vi "Route Triggers Gain Ranging.vi"(0 "pxi trigger bus configuration [channel]":T1[](array[typedef]), 1 "scope":string, 2 "map(T)/unmap(F)":bool=TRUE, 5 "routing mode":enum16{"Master Channel", "Independent Channels"}(ring), 11 "error in":errorcluster, 13 "gain config PXI triggers [channel]":string[][](array[combo])=[["None"], ["None"]], 14 "mmWave port config PXI trigger [channel]":string[](array[combo])=["None"]) -> (15 "error out":errorcluster)   [LabVIEW 2019]
uses:
  TypeDefs/PXI Trigger Bus Info.ctl
  <instrlib>/niMmWave/ni3620/Config/v1/Host/Public/Typedefs/PXI Trigger.ctl
  <vilib>/Instr/_visa.llb/VISA Unmap Trigger Trigger Source.ctl
  <instrlib>/niMmWave/ni3620/Config/v1/Host/niMmWave Config v1 Host.lvlib
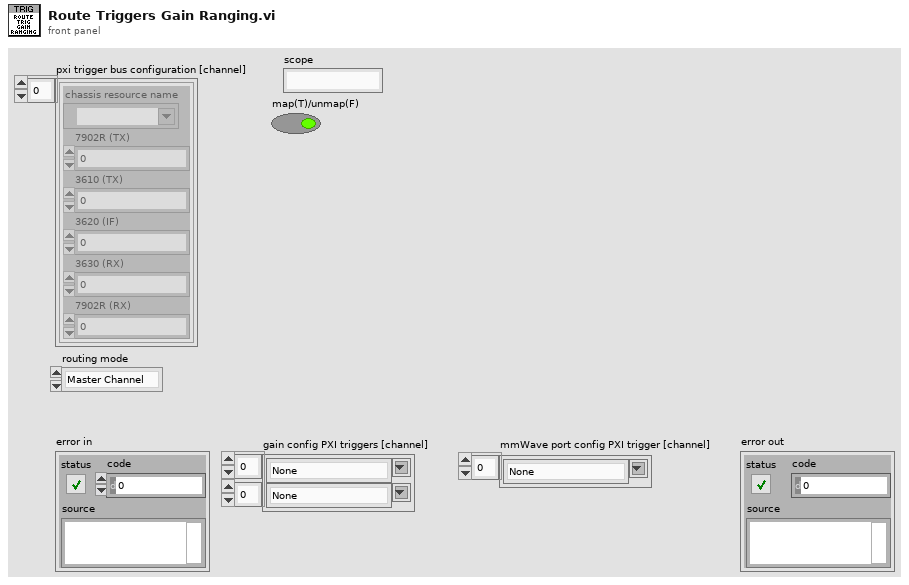
[diagram p1: front panel]
types:
  T1 = typedef "PXI Trigger Bus Info.ctl" = cluster{"chassis resource name":refnum<visa-resource-name>, "7902R (TX)":i16, "3610 (TX)":i16, "3620 (IF)":i16, "3630 (RX)":i16, "7902R (RX)":i16}
  T2 = typedef "niMmWave Config v1 Host.lvlib/PXI Trigger.ctl" = enum16{"PXI_Trig0", "PXI_Trig1", "PXI_Trig2", "PXI_Trig3", "PXI_Trig4", "PXI_Trig5", "PXI_Trig6", "PXI_Trig7", "None"}
  T3 = typedef "VISA Unmap Trigger Trigger Source.ctl" = i16
  T4 = cluster{"chassis":refnum<visa-resource-name>, "pxi trigger number":T3, "source trigger segment":i16, "destination trigger segment":i16}
  T5 = cluster{"chassis":refnum<visa-resource-name>, "pxi trigger number":T3, "source trigger segment":i16, "destination trigger segment":i16}[]
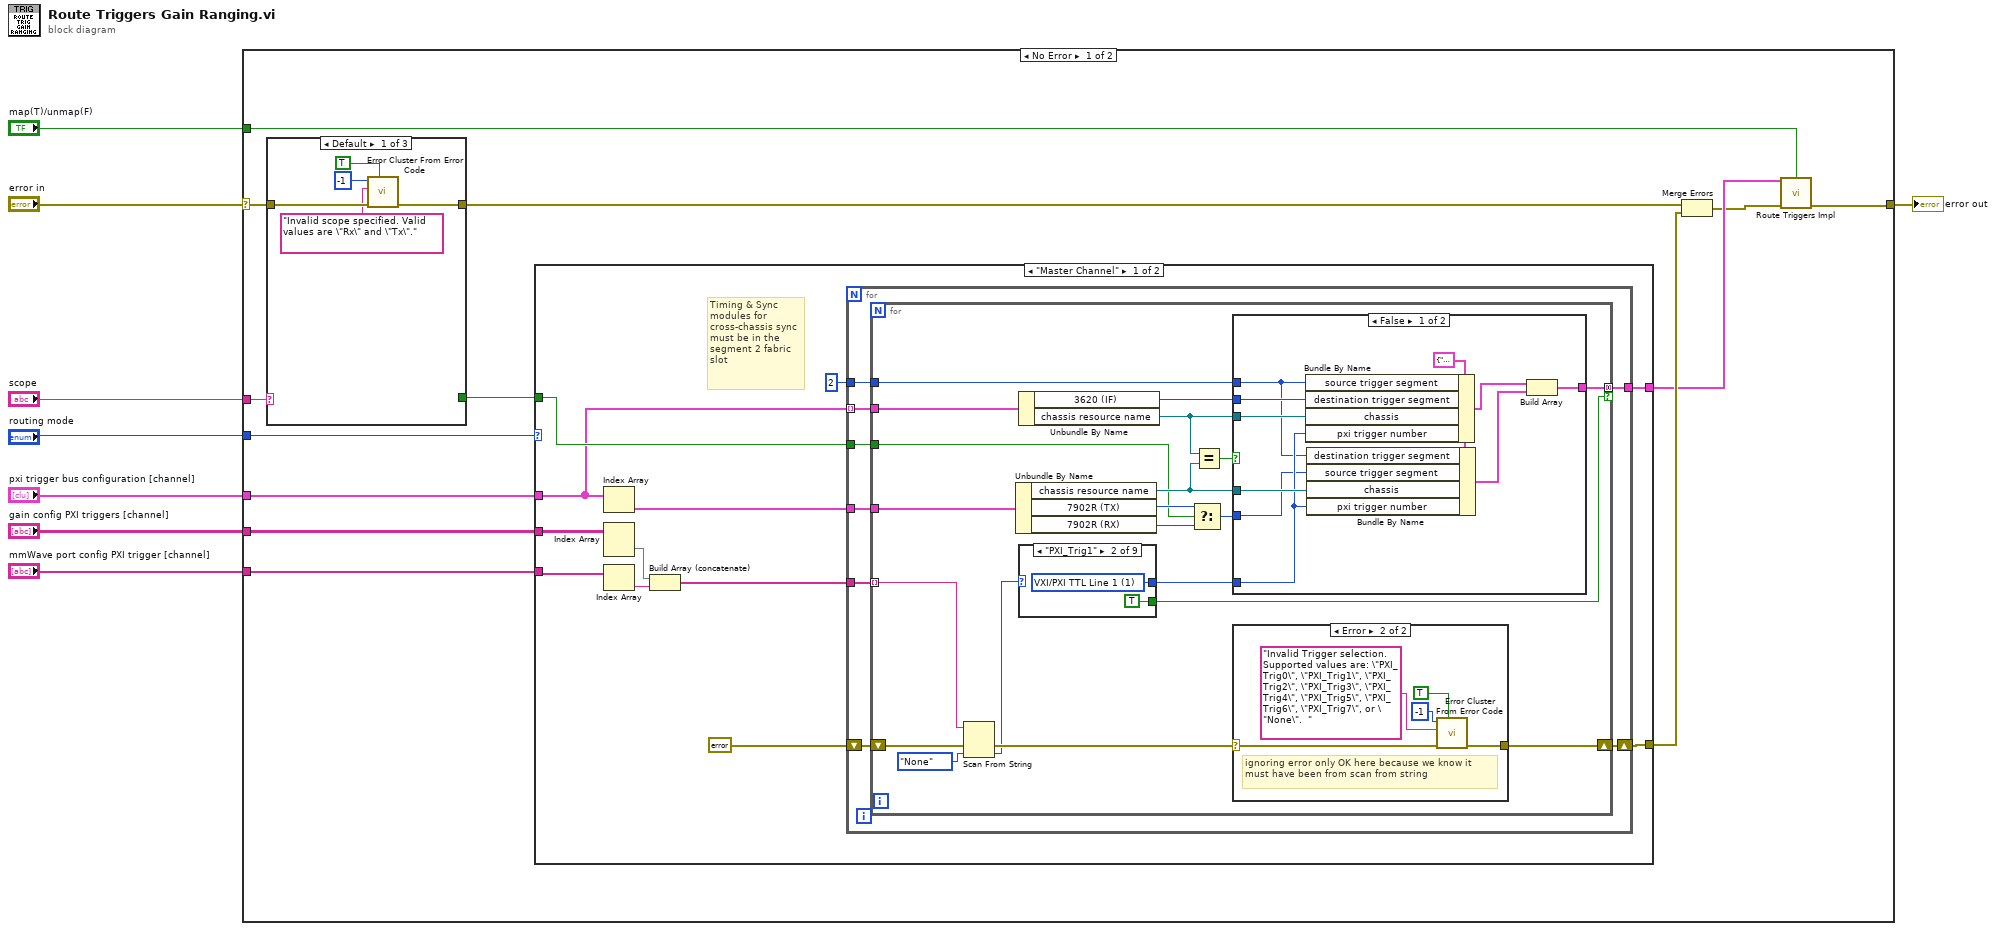
[diagram p0: block diagram]
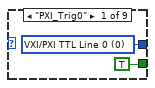
[diagram p3: hidden frame]
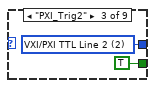
[diagram p4: hidden frame]
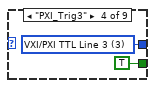
[diagram p5: hidden frame]
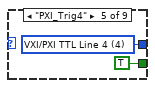
[diagram p6: hidden frame]
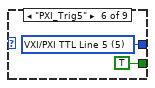
[diagram p7: hidden frame]
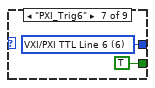
[diagram p8: hidden frame]
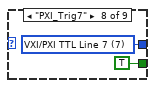
[diagram p9: hidden frame]
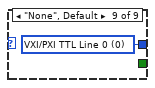
[diagram p10: hidden frame]
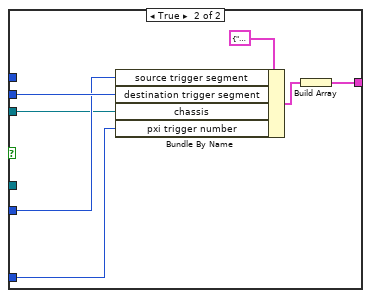
[diagram p11: hidden frame]
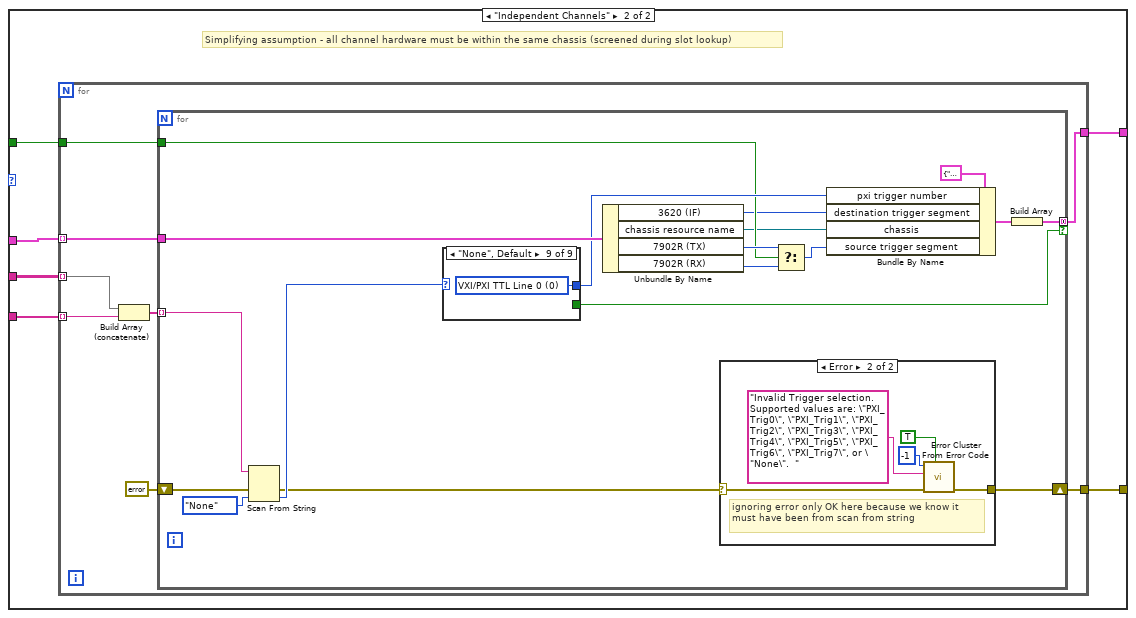
[diagram p12: hidden frame]
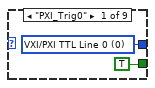
[diagram p14: hidden frame]
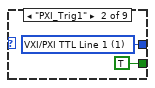
[diagram p15: hidden frame]
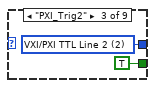
[diagram p16: hidden frame]
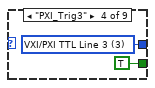
[diagram p17: hidden frame]
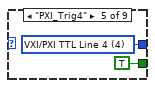
[diagram p18: hidden frame]
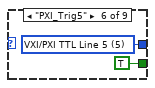
[diagram p19: hidden frame]
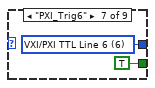
[diagram p20: hidden frame]
diagram:
  n1 = case shown="No Error" "error in" {
    selector: "error in" -> [w20 w166]
    tunnel: [w9 w166] -> w8
    tunnel: "map(T)/unmap(F)" -> [w11 _]
    tunnel: "pxi trigger bus configuration [channel]" -> [w21 _]
    tunnel: "scope" -> [w19 _]
    tunnel: "routing mode" -> [w17 _]
    tunnel: "gain config PXI triggers [channel]" -> [w16 _]
    tunnel: "mmWave port config PXI trigger [channel]" -> [w15 _]
    frame No Error {
      n2 = case shown="Default" w19 {
        tunnel: [w160 w163 w165] -> w14
        tunnel: w20 -> [w161 w163 w165]
        tunnel: [_ FALSE TRUE] -> w18
        frame Default {
          n3 = call <vilib>:"Error Cluster From Error Code.vi"("show call chain? (False)"=TRUE, "error in (no error)"=w161, "error message (\"\")"="Invalid scope specified. Valid values are \"Rx\" and \"Tx\"." ("error message (\"\")"), "error code (0)"=-1) -> ("error out"=w160:errorcluster)  [unwired: 5 in]
        }
        frame "rx" {
        }
        frame "tx" {
        }
      }
      n4 = case shown="\"Master Channel\"" w17 {
        tunnel: w21 -> [w22 w107]
        tunnel: [w33 w106] -> w12
        tunnel: w18 -> [w32 w105]
        tunnel: w16 -> [w29 w104]
        tunnel: w15 -> [w30 w103]
        tunnel: [w23 w102] -> w13
        frame "Master Channel" {
          # "Timing & Sync modules for cross-chassis sync must be in the segment 2 fabric slot"
          n5 = Index Array(array=w22) -> (element=w28:T1)  [unwired: 1 in]
          n6 = Index Array(array=w29) -> (element=w27:string[])  [unwired: 2 in]
          n7 = Index Array(array=w30) -> (element=w26:string)  [unwired: 1 in]
          n8 = Build Array (concatenate)(w27, w26) -> (w25:string[])
          n9 = for {
            tunnel: [w41] -> w33
            tunnel: w32 -> [w40]
            tunnel: i16 2 ("source trigger segment") -> [w39]
            tunnel: w28 -> [w38]
            tunnel: w25 -> [w37]
            tunnel: w22 -> [w34] mode=indexing
            shift-right: [w35] -> w23
            shift-left: errorcluster {"status"=FALSE, "code"=0, "source"=""} ("error out") -> [w36]
            n10 = for {
              tunnel: [w61] -> w41 mode=concatenating if=w43
              tunnel: w40 -> [w53]
              tunnel: w39 -> [w52]
              tunnel: w38 -> [w51]
              tunnel: w37 -> [w47] mode=indexing
              shift-right: [w45] -> w35
              shift-left: w36 -> [w46]
              tunnel: w34 -> [w42]
              n11 = Scan From String(input string=w47, error in=w46, default 1=PXI_Trigger."None" ("PXI Trigger")) -> (error out=w50:errorcluster, output 1=w49:T2)  [unwired: 2 in, 2 out]
              n12 = Unbundle By Name(w51) -> ("chassis resource name"=w59:refnum<visa-resource-name>, "7902R (TX)"=w56:i16, "7902R (RX)"=w55:i16)
              n13 = Unbundle By Name(w42) -> ("3620 (IF)"=w60:i16, "chassis resource name"=w57:refnum<visa-resource-name>)
              n14 = case shown="\"PXI_Trig1\"" w49 {
                tunnel: [w69 w71 w73 w75 w77 w79 w81 w83 w84] -> w44
                tunnel: [TRUE ("x = y?") TRUE ("x = y?") TRUE ("x = y?") TRUE ("x = y?") TRUE ("x = y?") TRUE ("x = y?") TRUE ("x = y?") TRUE ("x = y?") _] -> w43
                frame "PXI_Trig0" {
                  w69 = T3 0 items=["VXI/PXI TTL Line 0"=0, "VXI/PXI TTL Line 1"=1, "VXI/PXI TTL Line 2"=2, "VXI/PXI TTL Line 3"=3, "VXI/PXI TTL Line 4"=4, "VXI/PXI TTL Line 5"=5, "VXI/PXI TTL Line 6"=6, "VXI/PXI TTL Line 7"=7, "VXI ECL Line 0"=8, "VXI ECL Line 1"=9, "Front Panel Input"=27, "Front Panel Output"=28] ("pxi trigger number")
                }
                frame "PXI_Trig1" {
                  w71 = T3 1 items=["VXI/PXI TTL Line 0"=0, "VXI/PXI TTL Line 1"=1, "VXI/PXI TTL Line 2"=2, "VXI/PXI TTL Line 3"=3, "VXI/PXI TTL Line 4"=4, "VXI/PXI TTL Line 5"=5, "VXI/PXI TTL Line 6"=6, "VXI/PXI TTL Line 7"=7, "VXI ECL Line 0"=8, "VXI ECL Line 1"=9, "Front Panel Input"=27, "Front Panel Output"=28] ("pxi trigger number")
                }
                frame "PXI_Trig2" {
                  w73 = T3 2 items=["VXI/PXI TTL Line 0"=0, "VXI/PXI TTL Line 1"=1, "VXI/PXI TTL Line 2"=2, "VXI/PXI TTL Line 3"=3, "VXI/PXI TTL Line 4"=4, "VXI/PXI TTL Line 5"=5, "VXI/PXI TTL Line 6"=6, "VXI/PXI TTL Line 7"=7, "VXI ECL Line 0"=8, "VXI ECL Line 1"=9, "Front Panel Input"=27, "Front Panel Output"=28] ("pxi trigger number")
                }
                frame "PXI_Trig3" {
                  w75 = T3 3 items=["VXI/PXI TTL Line 0"=0, "VXI/PXI TTL Line 1"=1, "VXI/PXI TTL Line 2"=2, "VXI/PXI TTL Line 3"=3, "VXI/PXI TTL Line 4"=4, "VXI/PXI TTL Line 5"=5, "VXI/PXI TTL Line 6"=6, "VXI/PXI TTL Line 7"=7, "VXI ECL Line 0"=8, "VXI ECL Line 1"=9, "Front Panel Input"=27, "Front Panel Output"=28] ("pxi trigger number")
                }
                frame "PXI_Trig4" {
                  w77 = T3 4 items=["VXI/PXI TTL Line 0"=0, "VXI/PXI TTL Line 1"=1, "VXI/PXI TTL Line 2"=2, "VXI/PXI TTL Line 3"=3, "VXI/PXI TTL Line 4"=4, "VXI/PXI TTL Line 5"=5, "VXI/PXI TTL Line 6"=6, "VXI/PXI TTL Line 7"=7, "VXI ECL Line 0"=8, "VXI ECL Line 1"=9, "Front Panel Input"=27, "Front Panel Output"=28] ("pxi trigger number")
                }
                frame "PXI_Trig5" {
                  w79 = T3 5 items=["VXI/PXI TTL Line 0"=0, "VXI/PXI TTL Line 1"=1, "VXI/PXI TTL Line 2"=2, "VXI/PXI TTL Line 3"=3, "VXI/PXI TTL Line 4"=4, "VXI/PXI TTL Line 5"=5, "VXI/PXI TTL Line 6"=6, "VXI/PXI TTL Line 7"=7, "VXI ECL Line 0"=8, "VXI ECL Line 1"=9, "Front Panel Input"=27, "Front Panel Output"=28] ("pxi trigger number")
                }
                frame "PXI_Trig6" {
                  w81 = T3 6 items=["VXI/PXI TTL Line 0"=0, "VXI/PXI TTL Line 1"=1, "VXI/PXI TTL Line 2"=2, "VXI/PXI TTL Line 3"=3, "VXI/PXI TTL Line 4"=4, "VXI/PXI TTL Line 5"=5, "VXI/PXI TTL Line 6"=6, "VXI/PXI TTL Line 7"=7, "VXI ECL Line 0"=8, "VXI ECL Line 1"=9, "Front Panel Input"=27, "Front Panel Output"=28] ("pxi trigger number")
                }
                frame "PXI_Trig7" {
                  w83 = T3 7 items=["VXI/PXI TTL Line 0"=0, "VXI/PXI TTL Line 1"=1, "VXI/PXI TTL Line 2"=2, "VXI/PXI TTL Line 3"=3, "VXI/PXI TTL Line 4"=4, "VXI/PXI TTL Line 5"=5, "VXI/PXI TTL Line 6"=6, "VXI/PXI TTL Line 7"=7, "VXI ECL Line 0"=8, "VXI ECL Line 1"=9, "Front Panel Input"=27, "Front Panel Output"=28] ("pxi trigger number")
                }
                frame "None", Default {
                  w84 = T3 0 items=["VXI/PXI TTL Line 0"=0, "VXI/PXI TTL Line 1"=1, "VXI/PXI TTL Line 2"=2, "VXI/PXI TTL Line 3"=3, "VXI/PXI TTL Line 4"=4, "VXI/PXI TTL Line 5"=5, "VXI/PXI TTL Line 6"=6, "VXI/PXI TTL Line 7"=7, "VXI ECL Line 0"=8, "VXI ECL Line 1"=9, "Front Panel Input"=27, "Front Panel Output"=28] ("pxi trigger number")
                }
              }
              n15 = Select(t=w56, s=w53, f=w55) -> (s? t:f=w54:i16)
              n16 = Equal?(x=w57, y=w59) -> (x = y?=w58:bool)
              n17 = case shown="False" w58 {
                tunnel: [w93 w100] -> w61
                tunnel: w60 -> [w92 w98]
                tunnel: w59 -> [w89 _]
                tunnel: w57 -> [w91 w95]
                tunnel: w52 -> [w85 _]
                tunnel: w54 -> [w86 w97]
                tunnel: w44 -> [w87 w96]
                frame False {
                  w90 = T4 {"chassis"="", "pxi trigger number"=0, "source trigger segment"=0, "destination trigger segment"=0} ("Trigger Route")
                  n18 = Bundle By Name(cluster=w90, "source trigger segment"=w85, "destination trigger segment"=w92, "chassis"=w91, "pxi trigger number"=w87) -> (w94:T4)
                  n19 = Bundle By Name(cluster=w90, "destination trigger segment"=w85, "source trigger segment"=w86, "chassis"=w89, "pxi trigger number"=w87) -> (w88:T4)
                  n20 = Build Array(w94, w88) -> (w93:T5)
                }
                frame True {
                  n21 = Bundle By Name(cluster=T4 {"chassis"="", "pxi trigger number"=0, "source trigger segment"=0, "destination trigger segment"=0} ("Trigger Route"), "source trigger segment"=w97, "destination trigger segment"=w98, "chassis"=w95, "pxi trigger number"=w96) -> (w101:T4)
                  n22 = Build Array(w101) -> (w100:T5)
                }
              }
              n23 = case shown="Error" w50 {
                selector: w50 -> [w62 w63]
                tunnel: [w62 w64] -> w45
                frame No Error {
                }
                frame Error {
                  # "ignoring error only OK here because we know it must have been from scan from string"
                  n24 = call <vilib>:"Error Cluster From Error Code.vi"("show call chain? (False)"=TRUE, "error in (no error)"=w63, "error message (\"\")"="Invalid Trigger selection. Supported values are: \"PXI_Trig0\", \"PXI_Trig1\", \"PXI_Trig2\", \"PXI_Trig3\", \"PXI_Trig4\", \"PXI_Trig5\", \"PXI_Trig6\", \"PXI_Trig7\", or \"None\".  " ("error message (\"\")"), "error code (0)"=-1) -> ("error out"=w64:errorcluster)  [unwired: 5 in]
                }
              }
            }
          }
        }
        frame "Independent Channels" {
          # "Simplifying assumption - all channel hardware must be within the same chassis (screened during slot lookup)"
          n25 = for {
            tunnel: w107 -> [w115] mode=indexing
            tunnel: [w114] -> w106
            tunnel: w105 -> [w113]
            tunnel: w104 -> [w112] mode=indexing
            tunnel: w103 -> [w111] mode=indexing
            tunnel: [w109] -> w102
            n26 = Build Array (concatenate)(w112, w111) -> (w110:string[])
            n27 = for {
              tunnel: w110 -> [w133] mode=indexing
              tunnel: w115 -> [w128]
              tunnel: [w127] -> w114 mode=concatenating if=w125
              tunnel: w113 -> [w124]
              shift-right: [w117] -> w109
              shift-left: errorcluster {"status"=FALSE, "code"=0, "source"=""} ("error out") -> [w116]
              n28 = Scan From String(input string=w133, error in=w116, default 1=PXI_Trigger."None" ("PXI Trigger")) -> (error out=w118:errorcluster, output 1=w131:T2)  [unwired: 2 in, 2 out]
              n29 = case shown="\"None\", Default" w131 {
                tunnel: [w141 w143 w145 w147 w149 w151 w153 w155 w156] -> w126
                tunnel: [TRUE ("x = y?") TRUE ("x = y?") TRUE ("x = y?") TRUE ("x = y?") TRUE ("x = y?") TRUE ("x = y?") TRUE ("x = y?") TRUE ("x = y?") _] -> w125
                frame "PXI_Trig0" {
                  w141 = T3 0 items=["VXI/PXI TTL Line 0"=0, "VXI/PXI TTL Line 1"=1, "VXI/PXI TTL Line 2"=2, "VXI/PXI TTL Line 3"=3, "VXI/PXI TTL Line 4"=4, "VXI/PXI TTL Line 5"=5, "VXI/PXI TTL Line 6"=6, "VXI/PXI TTL Line 7"=7, "VXI ECL Line 0"=8, "VXI ECL Line 1"=9, "Front Panel Input"=27, "Front Panel Output"=28] ("pxi trigger number")
                }
                frame "PXI_Trig1" {
                  w143 = T3 1 items=["VXI/PXI TTL Line 0"=0, "VXI/PXI TTL Line 1"=1, "VXI/PXI TTL Line 2"=2, "VXI/PXI TTL Line 3"=3, "VXI/PXI TTL Line 4"=4, "VXI/PXI TTL Line 5"=5, "VXI/PXI TTL Line 6"=6, "VXI/PXI TTL Line 7"=7, "VXI ECL Line 0"=8, "VXI ECL Line 1"=9, "Front Panel Input"=27, "Front Panel Output"=28] ("pxi trigger number")
                }
                frame "PXI_Trig2" {
                  w145 = T3 2 items=["VXI/PXI TTL Line 0"=0, "VXI/PXI TTL Line 1"=1, "VXI/PXI TTL Line 2"=2, "VXI/PXI TTL Line 3"=3, "VXI/PXI TTL Line 4"=4, "VXI/PXI TTL Line 5"=5, "VXI/PXI TTL Line 6"=6, "VXI/PXI TTL Line 7"=7, "VXI ECL Line 0"=8, "VXI ECL Line 1"=9, "Front Panel Input"=27, "Front Panel Output"=28] ("pxi trigger number")
                }
                frame "PXI_Trig3" {
                  w147 = T3 3 items=["VXI/PXI TTL Line 0"=0, "VXI/PXI TTL Line 1"=1, "VXI/PXI TTL Line 2"=2, "VXI/PXI TTL Line 3"=3, "VXI/PXI TTL Line 4"=4, "VXI/PXI TTL Line 5"=5, "VXI/PXI TTL Line 6"=6, "VXI/PXI TTL Line 7"=7, "VXI ECL Line 0"=8, "VXI ECL Line 1"=9, "Front Panel Input"=27, "Front Panel Output"=28] ("pxi trigger number")
                }
                frame "PXI_Trig4" {
                  w149 = T3 4 items=["VXI/PXI TTL Line 0"=0, "VXI/PXI TTL Line 1"=1, "VXI/PXI TTL Line 2"=2, "VXI/PXI TTL Line 3"=3, "VXI/PXI TTL Line 4"=4, "VXI/PXI TTL Line 5"=5, "VXI/PXI TTL Line 6"=6, "VXI/PXI TTL Line 7"=7, "VXI ECL Line 0"=8, "VXI ECL Line 1"=9, "Front Panel Input"=27, "Front Panel Output"=28] ("pxi trigger number")
                }
                frame "PXI_Trig5" {
                  w151 = T3 5 items=["VXI/PXI TTL Line 0"=0, "VXI/PXI TTL Line 1"=1, "VXI/PXI TTL Line 2"=2, "VXI/PXI TTL Line 3"=3, "VXI/PXI TTL Line 4"=4, "VXI/PXI TTL Line 5"=5, "VXI/PXI TTL Line 6"=6, "VXI/PXI TTL Line 7"=7, "VXI ECL Line 0"=8, "VXI ECL Line 1"=9, "Front Panel Input"=27, "Front Panel Output"=28] ("pxi trigger number")
                }
                frame "PXI_Trig6" {
                  w153 = T3 6 items=["VXI/PXI TTL Line 0"=0, "VXI/PXI TTL Line 1"=1, "VXI/PXI TTL Line 2"=2, "VXI/PXI TTL Line 3"=3, "VXI/PXI TTL Line 4"=4, "VXI/PXI TTL Line 5"=5, "VXI/PXI TTL Line 6"=6, "VXI/PXI TTL Line 7"=7, "VXI ECL Line 0"=8, "VXI ECL Line 1"=9, "Front Panel Input"=27, "Front Panel Output"=28] ("pxi trigger number")
                }
                frame "PXI_Trig7" {
                  w155 = T3 7 items=["VXI/PXI TTL Line 0"=0, "VXI/PXI TTL Line 1"=1, "VXI/PXI TTL Line 2"=2, "VXI/PXI TTL Line 3"=3, "VXI/PXI TTL Line 4"=4, "VXI/PXI TTL Line 5"=5, "VXI/PXI TTL Line 6"=6, "VXI/PXI TTL Line 7"=7, "VXI ECL Line 0"=8, "VXI ECL Line 1"=9, "Front Panel Input"=27, "Front Panel Output"=28] ("pxi trigger number")
                }
                frame "None", Default {
                  w156 = T3 0 items=["VXI/PXI TTL Line 0"=0, "VXI/PXI TTL Line 1"=1, "VXI/PXI TTL Line 2"=2, "VXI/PXI TTL Line 3"=3, "VXI/PXI TTL Line 4"=4, "VXI/PXI TTL Line 5"=5, "VXI/PXI TTL Line 6"=6, "VXI/PXI TTL Line 7"=7, "VXI ECL Line 0"=8, "VXI ECL Line 1"=9, "Front Panel Input"=27, "Front Panel Output"=28] ("pxi trigger number")
                }
              }
              n30 = Unbundle By Name(w128) -> ("3620 (IF)"=w121:i16, "chassis resource name"=w120:refnum<visa-resource-name>, "7902R (TX)"=w129:i16, "7902R (RX)"=w130:i16)
              n31 = case shown="Error" w118 {
                selector: w118 -> [w134 w135]
                tunnel: [w134 w136] -> w117
                frame No Error {
                }
                frame Error {
                  # "ignoring error only OK here because we know it must have been from scan from string"
                  n32 = call <vilib>:"Error Cluster From Error Code.vi"("show call chain? (False)"=TRUE, "error in (no error)"=w135, "error message (\"\")"="Invalid Trigger selection. Supported values are: \"PXI_Trig0\", \"PXI_Trig1\", \"PXI_Trig2\", \"PXI_Trig3\", \"PXI_Trig4\", \"PXI_Trig5\", \"PXI_Trig6\", \"PXI_Trig7\", or \"None\".  " ("error message (\"\")"), "error code (0)"=-1) -> ("error out"=w136:errorcluster)  [unwired: 5 in]
                }
              }
              n33 = Select(t=w129, s=w124, f=w130) -> (s? t:f=w119:i16)
              n34 = Bundle By Name(cluster=T4 {"chassis"="", "pxi trigger number"=0, "source trigger segment"=0, "destination trigger segment"=0} ("Trigger Route"), "pxi trigger number"=w126, "destination trigger segment"=w121, "chassis"=w120, "source trigger segment"=w119) -> (w123:T4)
              n35 = Build Array(w123) -> (w127:T5)
            }
          }
        }
      }
      n36 = Merge Errors(w14, w13) -> (w10:errorcluster)
      n37 = call "Route Triggers Impl.vi"("trigger routes"=w12, "map(T)/unmap(F)"=w11, "error in"=w10) -> ("error out"=w9:errorcluster)  [unwired: 12 in]
    }
    frame Error {
    }
  }
  "error out" <- w8
